vi "Addmap.vi"(7 "LabVIEW Web Service Request":refnum<class "Web Request.lvclass">) -> (3 "value":string)   [LabVIEW 2014]
uses:
  <vilib>/wsapi/Web Request.lvclass
  Libraries/Map Data Folder/All-Lines.ctl
  Libraries/Map Data Folder/LineCluster.ctl
  Libraries/Map Data Folder/LineConnection.ctl
  Libraries/Map Data Folder/Map Data.lvlib
panel:
  out "rest of the binary string":string
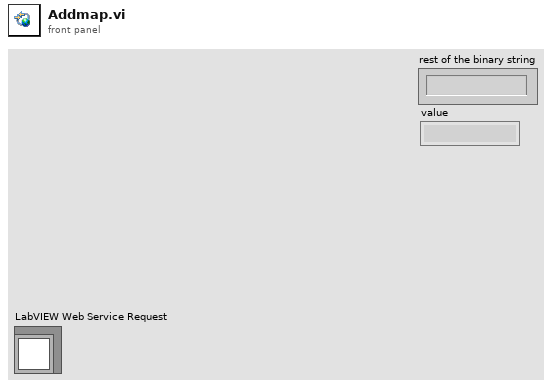
[diagram p1: front panel]
types:
  T1 = typedef "Map Data.lvlib/All-Lines.ctl" = T2[]
  T2 = typedef "Map Data.lvlib/LineCluster.ctl" = cluster{"Line name":string, "Line array":cluster{"X":dbl, "Y":dbl, "Z":dbl}[], "Line connections":T3[]}
  T3 = typedef "Map Data.lvlib/LineConnection.ctl" = cluster{"Index":i32, "Switch Pos":cluster{"X":dbl, "Y":dbl, "Z":dbl}, "Switch operational":bool, "Switch State":bool, "Connection Index":i32, "Connection Pos":cluster{"X":dbl, "Y":dbl, "Z":dbl}, "LinePos Index":i32, "ConnectPos Index":i32, "Same direction?":bool, "Manual Overide":bool, "Manual State":bool}
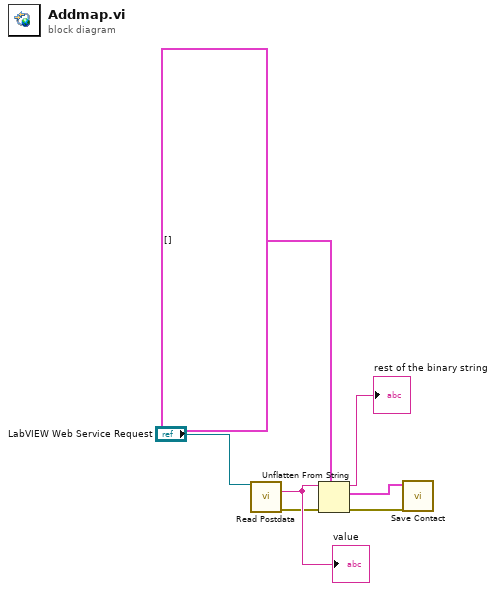
[diagram p0: block diagram]
diagram:
  n1 = call <vilib>:"Read Postdata.vi"("LabVIEW Web Service Request"="LabVIEW Web Service Request") -> ("postdata"=w5:string, "error out"=w4:errorcluster)  [unwired: 12 in, 1 out]
  "value" <- w5
  n2 = Unflatten From String(type=T1 [] ("All Lines"), binary string=w5, error in (no error)=w4) -> (rest of the binary string=→"rest of the binary string":string, value=w2:T1, error out=w7:errorcluster)  [unwired: 2 in]
  n3 = call "Save Contact.vi"("error in (no error)"=w7, "All Lines"=w2) -> ()  [unwired: 8 in, 2 out]
